vi "Datatype String to Datatype.vi"(11 "Datatype String":string) -> (3 "Generic Datatype":T1=enum."Bool")   [LabVIEW 2021, in "DataTypes_CIF_U.lvlib"]
doc: "Convert string names into generic datatype enum."
uses:
  DataTypes_CIF_U.lvlib
  Typedef/Generic Datatypes.ctl
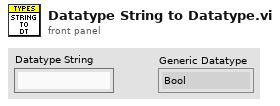
[diagram p1: front panel]
types:
  T1 = typedef "DataTypes_CIF_U.lvlib/Generic Datatypes.ctl" = enum16{"Invalid", "Bool", "U8", "I8", "U16", "I16", "U32", "I32", "U64", "I64", "Single Float", "Double Float", "String"}
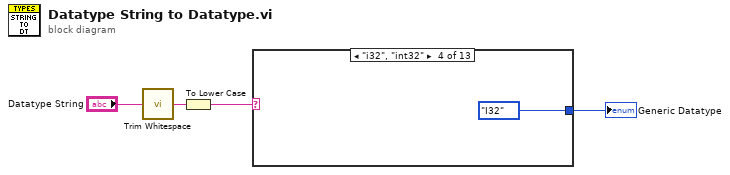
[diagram p0: block diagram]
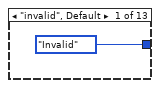
[diagram p2: hidden frame]
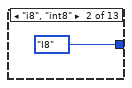
[diagram p3: hidden frame]
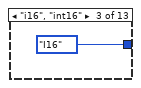
[diagram p4: hidden frame]
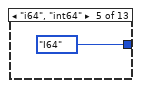
[diagram p5: hidden frame]
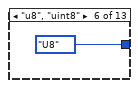
[diagram p6: hidden frame]
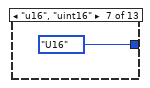
[diagram p7: hidden frame]
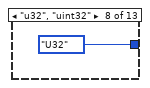
[diagram p8: hidden frame]
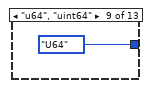
[diagram p9: hidden frame]
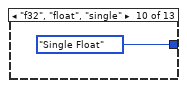
[diagram p10: hidden frame]
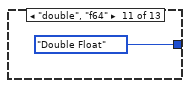
[diagram p11: hidden frame]
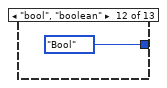
[diagram p12: hidden frame]
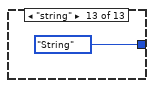
[diagram p13: hidden frame]
diagram:
  n1 = call <vilib>:"Trim Whitespace.vi"("string"="Datatype String") -> ("trimmed string"=w2:string)  [unwired: 1 in]
  n2 = To Lower Case(string=w2) -> (all lower case string=w1:string)
  n3 = case shown="\"i32\", \"int32\"" w1 {
    tunnel: [Generic_Datatypes."Invalid" ("Generic Datatype") Generic_Datatypes."I8" ("Generic Datatype") Generic_Datatypes."I16" ("Generic Datatype") Generic_Datatypes."I32" ("Generic Datatype") Generic_Datatypes."I64" ("Generic Datatype") Generic_Datatypes."U8" ("Generic Datatype") Generic_Datatypes."U16" ("Generic Datatype") Generic_Datatypes."U32" ("Generic Datatype") Generic_Datatypes."U64" ("Generic Datatype") Generic_Datatypes."Single Float" ("Generic Datatype") Generic_Datatypes."Double Float" ("Generic Datatype") Generic_Datatypes."Bool" ("Generic Datatype") Generic_Datatypes."String" ("Generic Datatype")] -> w4
    frame "invalid", Default {
    }
    frame "i8", "int8" {
    }
    frame "i16", "int16" {
    }
    frame "i32", "int32" {
    }
    frame "i64", "int64" {
    }
    frame "u8", "uint8" {
    }
    frame "u16", "uint16" {
    }
    frame "u32", "uint32" {
    }
    frame "u64", "uint64" {
    }
    frame "f32", "float", "single" {
    }
    frame "double", "f64" {
    }
    frame "bool", "boolean" {
    }
    frame "string" {
    }
  }
  "Generic Datatype" <- w4
